vi "Event MessengerM_DialogHelp.vi"() -> ()   [LabVIEW 2020]
panel:
  out "String 2":string="Event Messenger : a channel that allows each Write operation to trigger an event in a specified Event Structure."
  out "Context Help":string
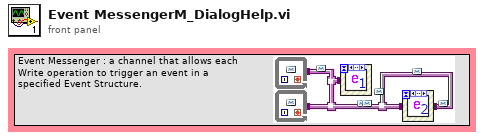
[diagram p1: front panel]
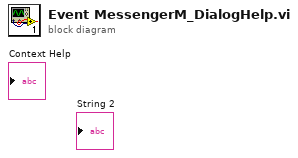
[diagram p0: block diagram]
diagram:
